vi "Insert Run Condition.vi"(8 "error in (no error)":errorcluster, 9 "狀態":enum16{"未連線", "運行中", "閒置", "故障"}(ring), 10 "device":i32=1, 11 "DBlink":string="Driver={ODBC Driver 17 for SQL Server};Server=localhost\\SQLEXPRESS;Database=YDXB01;UID=labview;PWD=123456789") -> (0 "error out":errorcluster)   [LabVIEW 2019]
uses:
  <vilib>/addons/database/Connection.llb/DB Tools Open Connec (String).vi
  <vilib>/addons/database/NI_Database_API.lvlib
panel:
  in  "狀態寫入":T1={"device_id"=2, "eqptstate"=0, "Time Stamp"=timestamp(0 s since 1904-01-01)}
  in  "columns":string[](array[string])=["device_id", "[sqptstate]", "create_time"]
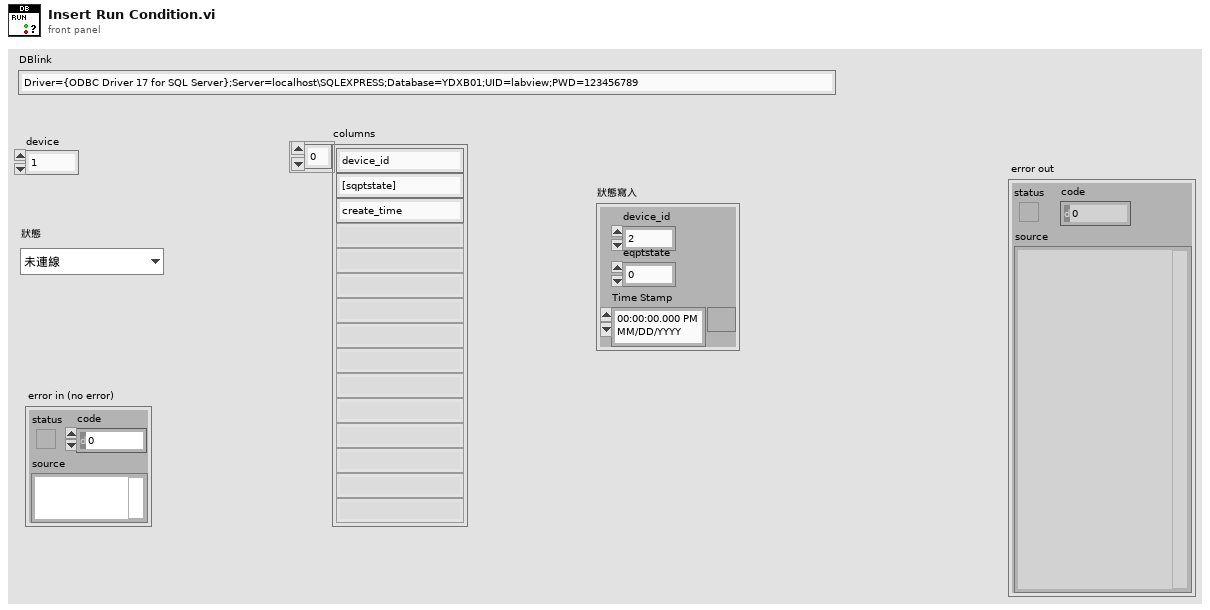
[diagram p1: front panel]
types:
  T1 = cluster{"device_id":i32, "eqptstate":i32, "Time Stamp":timestamp}
  T2 = typedef "NI_Database_API.lvlib/Conn ObjectReference.ctl" = refnum<k1>
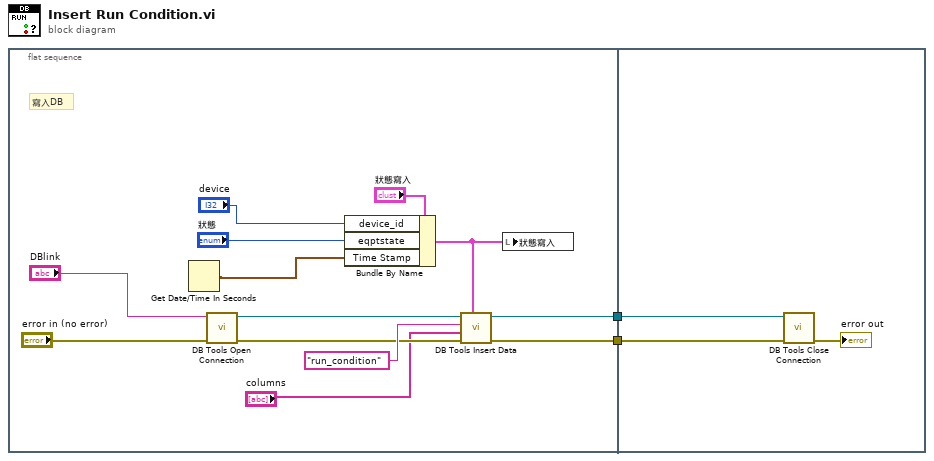
[diagram p0: block diagram]
diagram:
  n1 = flat-sequence {
    tunnel: [w13] -> w2
    tunnel: [w14] -> w1
    tunnel: w2 -> [w16]
    tunnel: w1 -> [w17]
    frame #0 {
      # "寫入DB"
      n2 = Get Date/Time In Seconds() -> (seconds since 1Jan1904=w3:timestamp)
      n3 = call-poly <vilib>:"DB Tools Open Connection.vi"("error in (no error)"="error in (no error)", "connection information"="DBlink") -> ("error out"=w11:errorcluster, "connection reference"=w10:T2)  [unwired: 6 in]
      n4 = Bundle By Name(cluster="狀態寫入", "device_id"="device", "eqptstate"="狀態", "Time Stamp"=w3) -> (w6:T1)
      n5 = call <vilib>:"DB Tools Insert Data.vi"("data"=w6, "error in (no error)"=w11, "columns"="columns", "table"="run_condition", "connection reference"=w10) -> ("error out"=w13:errorcluster, "connection reference out"=w14:T2)  [unwired: 5 in]
      n6 = local write "狀態寫入"(w6) -> ()
    }
    frame #1 {
      n7 = call <vilib>:"DB Tools Close Connection.vi"("error in (no error)"=w16, "connection reference"=w17) -> ("error out"=→"error out":errorcluster)  [unwired: 5 in]
    }
  }
